vi "NetConnectionsToServer.vi"(11 "Array":string[](array[string])=["net use \"\\\\nibataserver.apac.corp.natinst.com\\Reports\" /persistent:no /USER:apac.corp.natinst.com\\nibtest nibtest", "net use \"\\\\10.164.2.249\" /persistent:no /USER:apac\\nibtest nibtest", "net use \"\\\\in-ban-argo.natinst.com\" /persistent:no /USER:apac\\nibtest nibtest", "net use \"\\\\in-ban-argo\" /persistent:no /USER:apac\\nibtest nibtest"]) -> (0 "error out":errorcluster)   [LabVIEW 2013]
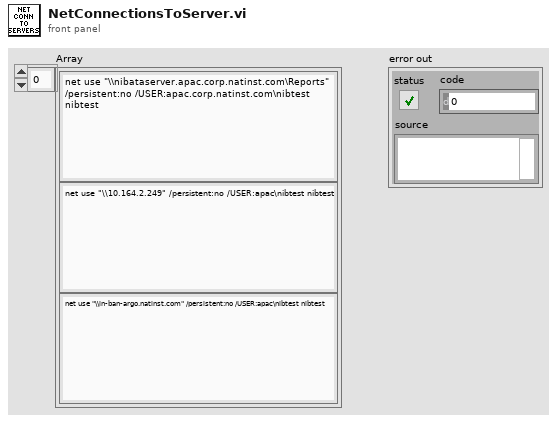
[diagram p1: front panel]
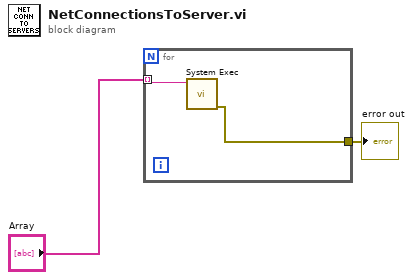
[diagram p0: block diagram]
diagram:
  n1 = for {
    tunnel: "Array" -> [w4] mode=indexing
    tunnel: [w3] -> w1
    n2 = call <vilib>:"System Exec.vi"("command line"=w4) -> ("error out"=w3:errorcluster)  [unwired: 7 in, 3 out]
  }
  "error out" <- w1
